vi "WLAN_FrameDetect.vi"(11 "input cluster":cluster{"t0":dbl, "dt":dbl, "Y":cdb[]}) -> (2 "is valid packet?":bool, 3 "output cluster":cluster{"t0":dbl, "dt":dbl, "Y":cdb[]})   [LabVIEW 2014]
uses:
  <vilib>/Analysis/2dsp.llb/1D Cross Correlation (CDB).vi
  <vilib>/Analysis/NI_AALPro.lvlib
panel:
  out "Waveform Graph 5":dbl[](graph)
  out "Waveform Graph 4":dbl[][](graph)
  out "Waveform Graph 3":dbl[][](graph)
  out "x-y":i32
  out "Waveform Graph 2":dbl[](graph)
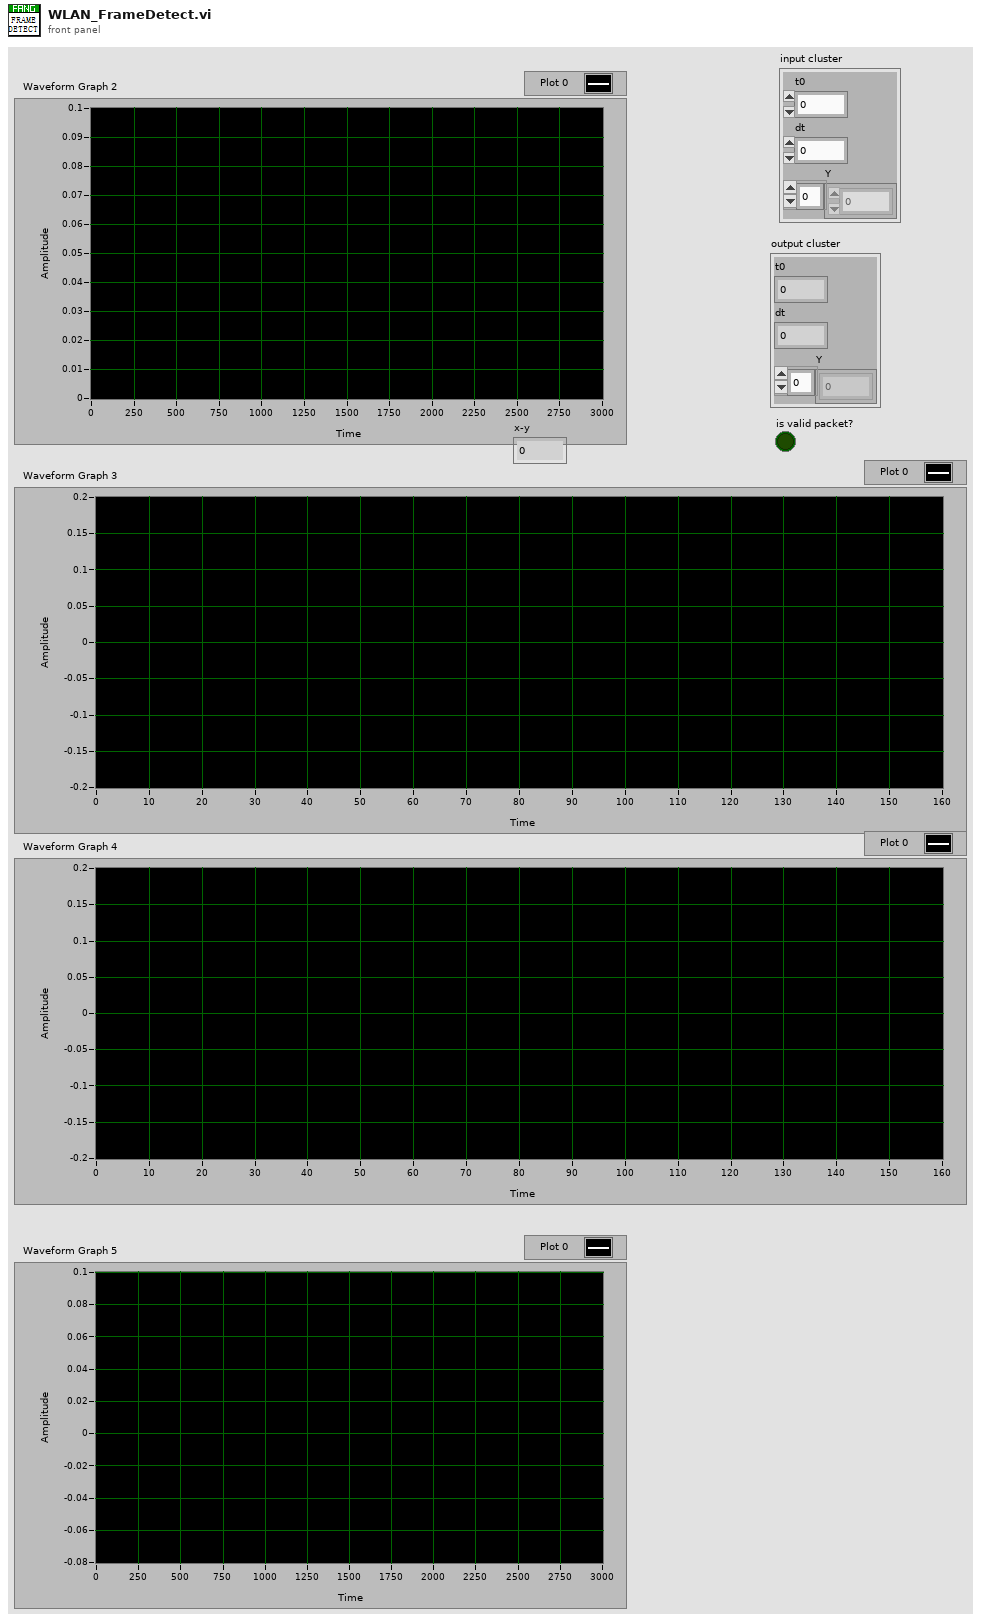
[diagram p1: front panel]
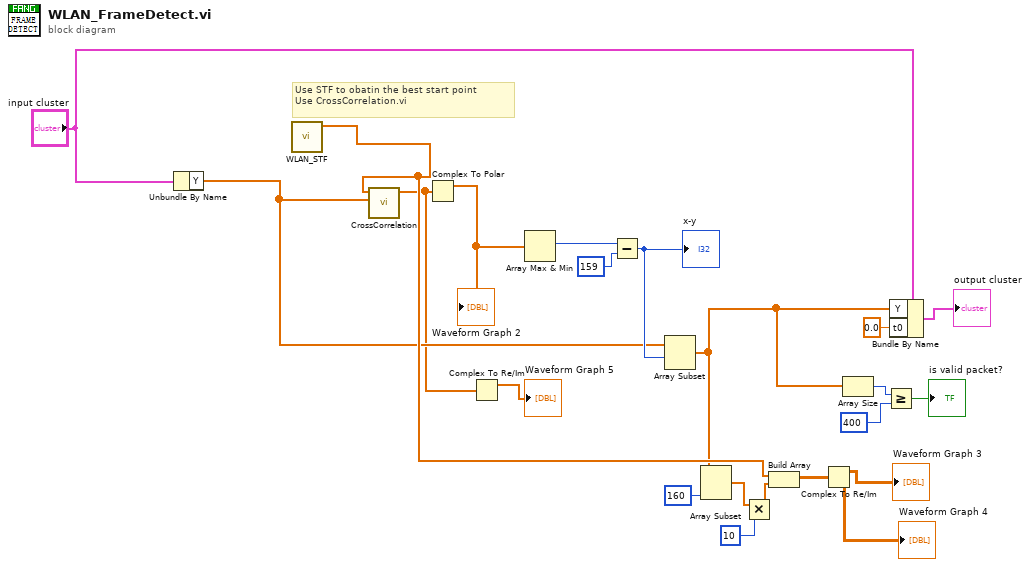
[diagram p0: block diagram]
diagram:
  # "Use STF to obatin the best start point\nUse CrossCorrelation.vi"
  n1 = Unbundle By Name("input cluster") -> ("Y"=w7:cdb[])
  n2 = call "WLAN_STF.vi"() -> ("STF"=w14:cdb[])  [unwired: 11 in]
  n3 = call-poly <vilib>:"CrossCorrelation.vi"("Y"=w7, "X"=w14) -> ("Rxy"=w2:cdb[])  [unwired: 8 in, 1 out]
  n4 = Complex To Polar(r * e^(i*theta)=w2) -> (r=w22:dbl[])  [unwired: 1 out]
  "Waveform Graph 2" <- w22
  n5 = Complex To Re/Im(x + iy=w2) -> (x=→"Waveform Graph 5":dbl[])  [unwired: 1 out]
  n6 = Array Max & Min(array=w22) -> (max index (indices)=w19:i32)  [unwired: 3 out]
  n7 = Subtract(x=w19, y=159) -> (x-y=w20:i32)
  "x-y" <- w20
  n8 = Array Subset(array=w7, index=w20) -> (w3:cdb[])  [unwired: 1 in]
  n9 = Array Subset(array=w3, length=160) -> (w13:cdb[])  [unwired: 1 in]
  n10 = Multiply(x=w13, y=10 ("length")) -> (x*y=w11:cdb[])
  n11 = Build Array(w14, w11) -> (w10:cdb[][])
  n12 = Complex To Re/Im(x + iy=w10) -> (x=→"Waveform Graph 3":dbl[][], y=→"Waveform Graph 4":dbl[][])
  n13 = Array Size(array=w3) -> (size(s)=w6:i32)
  n14 = Greater Or Equal?(x=w6, y=400) -> (x >= y?=→"is valid packet?":bool)
  n15 = Bundle By Name(cluster="input cluster", "Y"=w3, "t0"=0.0) -> (→"output cluster":cluster{"t0":dbl, "dt":dbl, "Y":cdb[]})
